vi "Write array to Config file.vi"(7 "section":string, 8 "error in (no error)":errorcluster, 9 "Array":string[](array[string]), 10 "key":string, 11 "Refnum in":T1) -> (0 "error out":errorcluster, 3 "refnum out":T1)   [LabVIEW 2015, in "SLSC Switch.lvlib" / "SLSC Switch.lvclass"]
uses:
  SLSC Switch.lvclass
  <vilib>/Utility/config.llb/Config Data RefNum.ctl
  <vilib>/Utility/config.llb/Write Key (String).vi
  <vilib>/Utility/config.llb/NI_LVConfig.lvlib
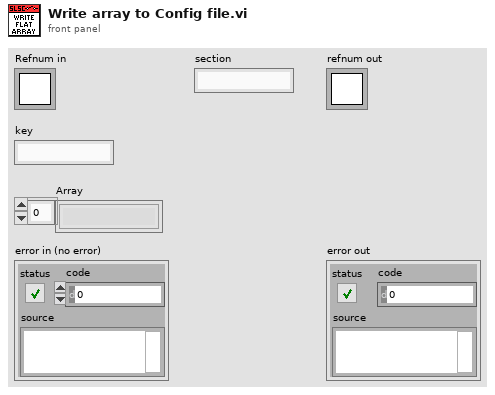
[diagram p1: front panel]
types:
  T1 = typedef "NI_LVConfig.lvlib/Config Data RefNum.ctl" = refnum<k1>
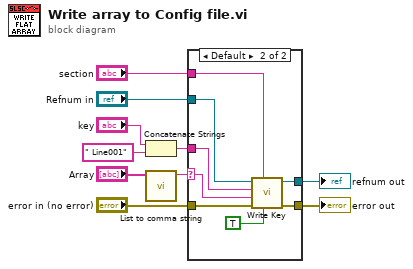
[diagram p0: block diagram]
diagram:
  n1 = Concatenate Strings("key", " Line001" ("string")) -> (w9:string)
  n2 = call "List to comma string.vi"("Array"="Array") -> ("String"=w3:string)  [unwired: 10 in]
  n3 = case shown="Default" w3 {
    selector: w3 -> [_ w20]
    tunnel: "Refnum in" -> [w12 w19]
    tunnel: "error in (no error)" -> [w11 w18]
    tunnel: [w12 w17] -> w1
    tunnel: [w11 w16] -> w2
    tunnel: w9 -> [_ w15]
    tunnel: "section" -> [_ w14]
    frame "" {
    }
    frame Default {
      n4 = call-poly <vilib>:"Write Key.vi"("write raw string? (F)"=TRUE, "section"=w14, "error in (no error)"=w18, "value"=w20, "key"=w15, "refnum"=w19) -> ("error out"=w16:errorcluster, "refnum out"=w17:T1)  [unwired: 3 in, 1 out]
    }
  }
  "error out" <- w2
  "refnum out" <- w1
